vi "Actor Core.vi"(8 "error in":errorcluster, 11 "CS++DIM-Client in":refnum<class "CS++DIM-Client.lvclass">) -> (0 "error out":errorcluster, 3 "Actor out":refnum<class "Actor.lvclass">)   [LabVIEW 2014, in "CS++DIM-Client.lvlib" / "CS++DIM-Client.lvclass"]
doc: "(<B>Filename</B>: Actor Framework.lvlib:Actor.lvclass:Actor Core.vi)\n\nReceives messages to the actor, reacts to them, and initiates any error handling that may shut the actor down.\n\nDescendant classes may override this VI to append parallel tasks for the actor to complete while it handles messages. Overrides use the Call Parent Method node."
uses:
  CS++DIM-Client.lvclass
  CSPP_Core/Actors/CS++GUIActor/CS++GUIActor.lvclass
  <vilib>/ActorFramework/Actor/Actor.lvclass
  CSPP_Core/Actors/CS++PVMonitor Messages/Register PVs Msg/Register PVs Msg.lvclass
  CSPP_Core/Actors/CS++BaseActor/CS++BaseActor.lvclass
  <vilib>/ActorFramework/Stop Msg/Stop Msg.lvclass
  DIM_Monitor/CS++DIMMonitor.lvclass
  CSPP_Core/Classes/CS++ProcessVariables/ProcessVariable/PV.lvclass
  CSPP_Core/Actors/CS++PVMonitor Messages/CS++PVUpdate Msg/CS++PVUpdate Msg.lvclass
  CSPP_Core/Actors/CS++GUIActor Messages/Update-PV Msg/Update-PV Msg.lvclass
panel:
  out "Data":T1(array[cluster])
  out "Last Update":timestamp
  in  "PV-Data":T2
  in  "Stop Button":bool
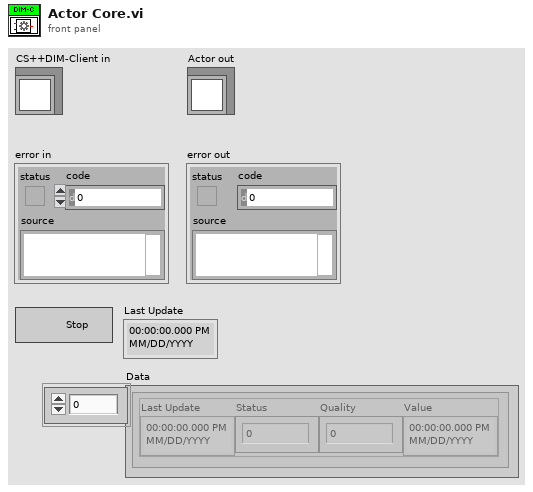
[diagram p1: front panel]
types:
  T1 = cluster{"Last Update":timestamp, "Status":i32, "Quality":i32, "Value":timestamp}[]
  T2 = cluster{"Last Update":timestamp, "Status":i32, "Quality":i32, "Value":timestamp}
  T3 = enum32{"Invalid", "Standard", "Closed", "Hidden", "Minimized", "Maximized"}
  T4 = cluster{"Self Enqueuer":refnum<class "Message Enqueuer.lvclass">, refnum<class "Update-PV Msg.lvclass">[]}
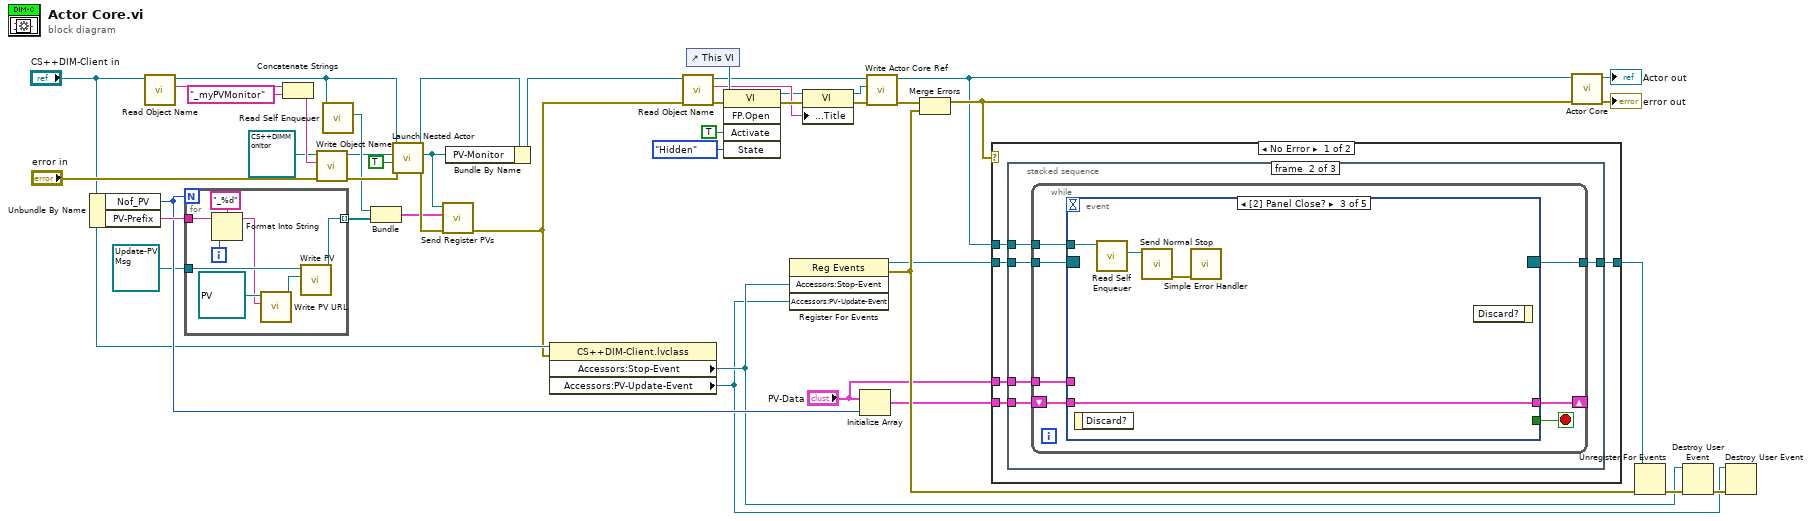
[diagram p0: block diagram]
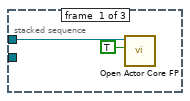
[diagram p2: hidden frame]
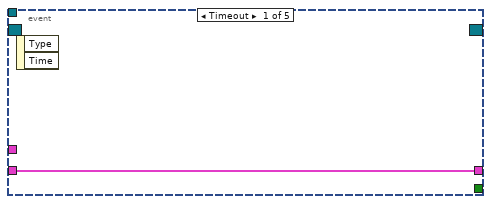
[diagram p3: hidden frame]
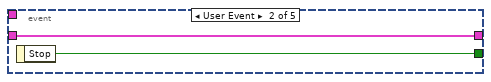
[diagram p4: hidden frame]
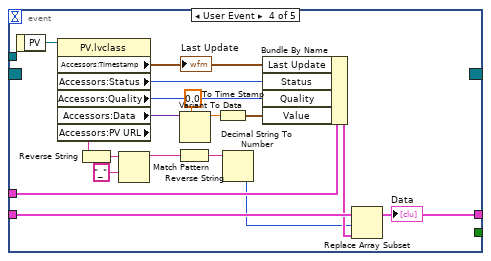
[diagram p5: hidden frame]
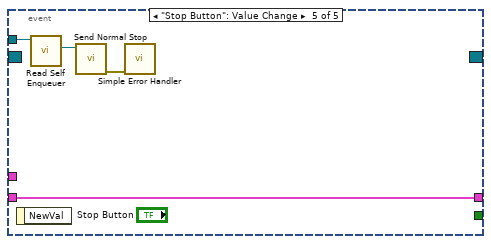
[diagram p6: hidden frame]
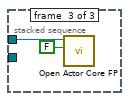
[diagram p7: hidden frame]
diagram:
  n1 = Unbundle By Name("CS++DIM-Client in") -> ("Nof_PV"=w15:i32, "PV-Prefix"=w25:string)
  n2 = call "Read Object Name.vi"("CS++BaseActor in"="CS++DIM-Client in") -> ("Object Name"=w32:string, "CS++BaseActor out"=w23:refnum<class "CS++DIM-Client.lvclass">)  [unwired: 8 in, 1 out]
  n3 = for {
    N: w15 -> [_]
    tunnel: w25 -> [w53]
    tunnel: [w46] -> w16 mode=indexing
    tunnel: refnum<class "Update-PV Msg.lvclass"> refnum ("CS++GUIActor.lvlib:Update-PV Msg.lvclass") -> [w48]
    i -> [w52]
    n4 = Format Into String(format string="_%d", initial string=w53, w52) -> (resulting string=w47:string)  [unwired: 1 in, 1 out]
    n5 = call "Write PV URL.vi"("PV URL"=w47, "PV in"=refnum<class "PV.lvclass"> refnum) -> ("PV out"=w49:refnum<class "PV.lvclass">)  [unwired: 8 in, 1 out]
    n6 = call "Write PV.vi"("PV"=w49, "CS++PVUpdate Msg in"=w48) -> ("CS++PVUpdate Msg out"=w46:refnum<class "Update-PV Msg.lvclass">)  [unwired: 8 in, 1 out]
  }
  n7 = Concatenate Strings(w32, "_myPVMonitor" ("Object Name")) -> (w30:string)
  n8 = call "Write Object Name.vi"("error in (no error)"="error in", "Object Name"=w30, "CS++BaseActor in"=refnum<class "CS++DIMMonitor.lvclass"> refnum ("CS++DIMMonitor.lvlib:CS++DIMMonitor.lvclass")) -> ("error out"=w27:errorcluster, "CS++BaseActor out"=w24:refnum<class "CS++DIMMonitor.lvclass">)  [unwired: 7 in]
  n9 = call <vilib>:"Read Self Enqueuer.vi"("Actor"=w23) -> ("Self Enqueuer"=w26:refnum<class "Message Enqueuer.lvclass">)  [unwired: 10 in]
  n10 = Bundle("Self Enqueuer"=w26, w16) -> (w43:T4)  [unwired: 1 in]
  n11 = call <vilib>:"Launch Nested Actor.vi"("error in (no error)"=w27, "Auto-stop? (T)"=TRUE, "Nested Actor"=w24, "Caller Actor in"=w23) -> ("error out"=w45:errorcluster, "Nested Actor's Enqueuer"=w44:refnum<class "Message Enqueuer.lvclass">, "Caller Actor out"=w22:refnum<class "CS++DIM-Client.lvclass">)  [unwired: 5 in]
  n12 = call "Send Register PVs.vi"("error in (no error)"=w45, "Register Info"=w43, "Message Enqueuer"=w44) -> ("error out"=w8:errorcluster)  [unwired: 7 in, 1 out]
  n13 = Bundle By Name(cluster=w22, "PV-Monitor"=w44) -> (w12:refnum<class "CS++DIM-Client.lvclass">)
  n14 = property class="CS++DIM-Client.lvclass"(reference="CS++DIM-Client in", error in=w8) -> ("Accessors:Stop-Event"=w10:refnum<user-event>, "Accessors:PV-Update-Event"=w9:refnum<user-event>)  [unwired: 2 out]
  n15 = call "Read Object Name.vi"("error in (no error)"=w8, "CS++BaseActor in"=w12) -> ("error out"=w7:errorcluster, "Object Name"=w38:string, "CS++BaseActor out"=w5:refnum<class "CS++DIM-Client.lvclass">)  [unwired: 7 in]
  n16 = control-ref of="This VI"() -> (w42:refnum<vi>)
  n17 = invoke class="VI" method="FP.Open"(reference=w42, error in=w7, "Activate"=TRUE ("Activate?"), "State"=T3."Hidden") -> (reference out=w33:refnum<vi>, error out=w39:errorcluster)  [unwired: 1 in, 3 out]
  n18 = register-events(w10, w9) -> (reference out=w35:refnum<event-registration>, error out=w36:errorcluster)  [unwired: 2 in]
  n19 = property class="VI"(reference=w33, error in=w39, "Front Panel.Title"=w38) -> (reference out=w1:refnum<vi>, error out=w3:errorcluster)
  n20 = Initialize Array("PV-Data", w15) -> (w14:T1)
  n21 = call "Write Actor Core Ref.vi"("error in (no error)"=w3, "Actor Core Ref"=w1, "CS++BaseActor in"=w5) -> ("error out"=w2:errorcluster, "CS++BaseActor out"=w4:refnum<class "CS++DIM-Client.lvclass">)  [unwired: 7 in]
  n22 = Merge Errors(w2, w36) -> (w29:errorcluster)
  n23 = case shown="No Error" w29 {
    tunnel: w4 -> [w58 _]
    tunnel: w35 -> [w57 w104]
    tunnel: [w56 w104] -> w34
    tunnel: w14 -> [w55 _]
    tunnel: "PV-Data" -> [w54 _]
    frame No Error {
      n24 = stacked-sequence {
        tunnel: w58 -> [w60 w64 w103]
        tunnel: w57 -> [_ w65 _]
        tunnel: [_ w63 _] -> w56
        tunnel: w55 -> [_ w62 _]
        tunnel: w54 -> [_ w61 _]
        frame #0 {
          n25 = call "Open Actor Core FP.vi"("Open FP (F)"=TRUE, "CS++BaseActor in"=w60) -> ()  [unwired: 8 in, 2 out]
        }
        frame #1 {
          n26 = while {
            tunnel: w65 -> [w72]
            tunnel: w64 -> [w71]
            tunnel: [w69] -> w63
            shift-right: [w66] -> _
            shift-left: w62 -> [w68]
            tunnel: w61 -> [w67]
            stop <- w70 stop-if-true
            n27 = event shown="[2] Panel Close?" {
              selector: w72 -> [_ _ _ _ _]
              dyn-events: [_ _ _ _ _] -> w69
              timeout: _ -> [_ _ _ _ _]
              tunnel: w71 -> [_ _ w77 _ w101]
              tunnel: [_ w75 _ _ _] -> w70
              tunnel: w68 -> [w73 w74 w76 w88 w98]
              tunnel: w67 -> [_ _ _ w93 _]
              tunnel: [w73 w74 w76 w87 w98] -> w66
              event Timeout {
                n28 = event-data() -> ()  [unwired: 1 in, 2 out]
              }
              event User Event {
                n29 = event-data() -> ("Stop"=w75:bool)  [unwired: 1 in]
              }
              event Panel Close? {
                n30 = event-data() -> ()  [unwired: 1 in, 1 out]
                n31 = call <vilib>:"Read Self Enqueuer.vi"("Actor"=w77) -> ("Self Enqueuer"=w79:refnum<class "Message Enqueuer.lvclass">)  [unwired: 10 in]
                n32 = call <vilib>:"Send Normal Stop.vi"("Message Enqueuer"=w79) -> ("error out"=w78:errorcluster)  [unwired: 10 in]
                n33 = call <vilib>:"Simple Error Handler.vi"("error in (no error)"=w78) -> ()  [unwired: 4 in, 5 out]
                n34 = event-data() -> ()  [unwired: 2 in, 1 out]
              }
              event User Event {
                n35 = event-data() -> ("PV"=w97:refnum<class "PV.lvclass">)  [unwired: 1 in]
                n36 = property class="PV.lvclass"(reference=w97) -> ("Accessors:Timestamp"=w92:timestamp, "Accessors:Status"=w91:i32, "Accessors:Quality"=w90:i32, "Accessors:Data"=w96:variant, "Accessors:PV URL"=w85:string)  [unwired: 1 in, 2 out]
                "Last Update" <- w92
                n37 = Reverse String(1:w85) -> (0:w84:string)
                n38 = Match Pattern(string=w84, regular expression="_") -> (before substring=w82:string)  [unwired: 1 in, 3 out]
                n39 = Reverse String(1:w82) -> (0:w81:string)
                n40 = Variant To Data(type=0.0, Variant=w96) -> (data=w94:dbl)  [unwired: 1 in, 1 out]
                n41 = To Time Stamp(1:w94) -> (0:w89:timestamp)
                n42 = Decimal String To Number(string=w81) -> (number=w80:i32)  [unwired: 2 in, 1 out]
                n43 = Bundle By Name(cluster=w93, "Last Update"=w92, "Status"=w91, "Quality"=w90, "Value"=w89) -> (w86:T2)
                n44 = Replace Array Subset(array=w88, new element=w86, index=w80) -> (w87:T1)
                "Data" <- w87
              }
              event "Stop Button": Value Change {
                n45 = event-data() -> ()  [unwired: 1 in, 1 out]
                n46 = call <vilib>:"Read Self Enqueuer.vi"("Actor"=w101) -> ("Self Enqueuer"=w100:refnum<class "Message Enqueuer.lvclass">)  [unwired: 10 in]
                n47 = call <vilib>:"Send Normal Stop.vi"("Message Enqueuer"=w100) -> ("error out"=w99:errorcluster)  [unwired: 10 in]
                n48 = call <vilib>:"Simple Error Handler.vi"("error in (no error)"=w99) -> ()  [unwired: 4 in, 5 out]
              }
            }
          }
        }
        frame #2 {
          n49 = call "Open Actor Core FP.vi"("Open FP (F)"=FALSE, "CS++BaseActor in"=w103) -> ()  [unwired: 8 in, 2 out]
        }
      }
    }
    frame Error {
    }
  }
  n50 = call-parent "Actor Core.vi"("error in"=w29, "CS++GUIActor in"=w4) -> ("error out"=→"error out":errorcluster, "Actor out"=→"Actor out":refnum<class "Actor.lvclass">)  [unwired: 8 in]
  n51 = Unregister For Events(event registration refnum=w34, error in=w36) -> (error out=w37:errorcluster)
  n52 = Destroy User Event(user event=w10, error in=w37) -> (error out=w28:errorcluster)
  n53 = Destroy User Event(user event=w9, error in=w28) -> ()  [unwired: 1 out]
